vi "Command Engine.vi"(8 "error in (no error)":errorcluster, 10 "Parameters":T1 {"Config"."Industrial Settings"."Write Refs"."Data Reference" format="%.0x"; "Config"."Industrial Settings"."Read Refs"."Data Reference" format="%.0x"; "Config"."PID Settings"."Read Refs"."Data Reference" format="%.0x"; "Config"."PID Settings"."Write Refs"."Data Reference" format="%.0x"}, 11 "State Variables":T9) -> (0 "error out":errorcluster)   [LabVIEW 2015, in "Control Addon Engine.lvlib"]
uses:
  Control Addon Engine.lvlib
  Types/Network Engine State Variables.ctl
  <vilib>/NI/NI VeriStand Inline Async API/_VS Inline Async API/Process/Process.lvclass
  <vilib>/NI/VeriStand Addon Network Comm/Engine/VeriStand Comm.lvclass
  Types/RT Configuration.ctl
  Shared/Types/Gain Schedule.ctl
  Shared/Types/Compiled Settings.ctl
  Shared/Types/Compiled PID Settings.ctl
  <vilib>/NI Veristand/Custom Device API/Block Data Reference.ctl
  <vilib>/NI Veristand/Custom Device API/Data Reference.ctl
  Shared/Types/Compiled Industrial Settings.ctl
  Shared/Types/Compiled Industrial Parameters.ctl
  <vilib>/NI/VeriStand Addon Network Comm/Engine/VeriStand Comm.lvclass/VeriStand Comm.ctl
  Shared/Types/Update Parameters Message.ctl
  <vilib>/NI/NI VeriStand Inline Async API/_VS Inline Async API/Process/Process.lvclass/Process.ctl
  <vilib>/NI/NI VeriStand Inline Async API/_VS Inline Async API/Error Handling Process/SubVIs/Error.ConvertArray.vi
  <vilib>/NI/AMC/Read Next Message.vi
  <vilib>/NI/Tools/Keyed Array/Index.vi
  <vilib>/NI/AMC/Send Local Message.vi
  <vilib>/NI/AMC/Read Termination Message.vi
  <vilib>/NI/Tools/Keyed Array/Map String.vi
  <vilib>/NI/AMC/Create Single Message.vi
  <vilib>/NI/AMC/Update Message Routing Info.vi
  <vilib>/NI/Tools/String/Get Case Matching.vi
  <vilib>/NI/AMC/Send Message.vi
  <vilib>/NI/AMC/Globals.vi
  <vilib>/NI/VeriStand Addon Network Comm/Shared/Comm Constants.vi
  Shared/Control Addon Shared.lvlib
  <vilib>/NI VeriStand/Custom Device API/Custom Device API.lvlib
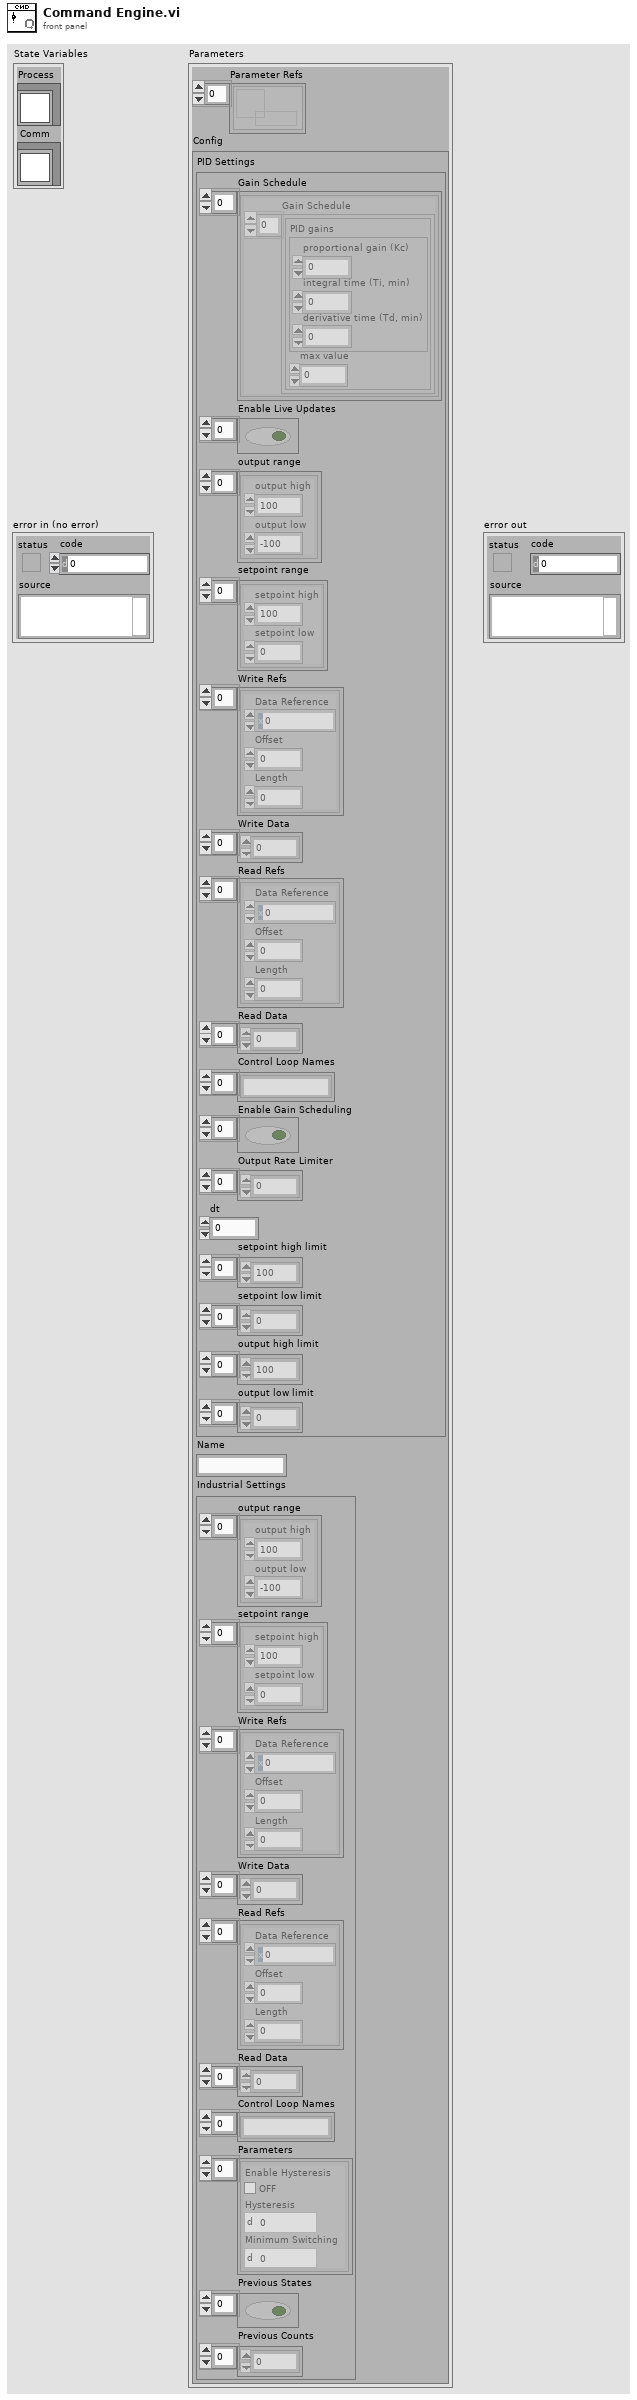
[diagram p1: front panel]
types:
  T1 = typedef "Control Addon Engine.lvlib/RT Configuration.ctl" = cluster{"Parameter Refs":refnum<data-value>[], "Config":T2}
  T2 = typedef "Control Addon Shared.lvlib/Compiled Settings.ctl" = cluster{"PID Settings":T3, "Name":string, "Industrial Settings":T7}
  T3 = typedef "Control Addon Shared.lvlib/Compiled PID Settings.ctl" = cluster{"Gain Schedule":T4[], "Enable Live Updates":bool[], "output range":cluster{"output high":dbl, "output low":dbl}[], "setpoint range":cluster{"setpoint high":dbl, "setpoint low":dbl}[], "Write Refs":T5[], "Write Data":dbl[], "Read Refs":T5[], "Read Data":dbl[], "Control Loop Names":string[], "Enable Gain Scheduling":bool[], "Output Rate Limiter":dbl[], "dt":dbl, "setpoint high limit":dbl[], "setpoint low limit":dbl[], "output high limit":dbl[], "output low limit":dbl[]}
  T4 = typedef "Control Addon Shared.lvlib/Gain Schedule.ctl" = cluster{"Gain Schedule":cluster{"PID gains":cluster{"proportional gain (Kc)":dbl, "integral time (Ti, min)":dbl, "derivative time (Td, min)":dbl}, "max value":dbl}[]}
  T5 = typedef "Custom Device API.lvlib/Block Data Reference.ctl" = cluster{"Data Reference":T6, "Offset":u64, "Length":u64}
  T6 = typedef "Custom Device API.lvlib/Data Reference.ctl" = i32
  T7 = typedef "Control Addon Shared.lvlib/Compiled Industrial Settings.ctl" = cluster{"output range":cluster{"output high":dbl, "output low":dbl}[], "setpoint range":cluster{"setpoint high":dbl, "setpoint low":dbl}[], "Write Refs":T5[], "Write Data":dbl[], "Read Refs":T5[], "Read Data":dbl[], "Control Loop Names":string[], "Parameters":T8[], "Previous States":bool[], "Previous Counts":u64[]}
  T8 = typedef "Control Addon Shared.lvlib/Compiled Industrial Parameters.ctl" = cluster{"Enable Hysteresis":bool, "Hysteresis":dbl, "Minimum Switching":u64}
  T9 = typedef "Control Addon Engine.lvlib/Network Engine State Variables.ctl" = cluster{"Process":refnum<class "Process.lvclass">, "Comm":refnum<class "VeriStand Comm.lvclass">}
  T10 = typedef "Control Addon Shared.lvlib/Update Parameters Message.ctl" = cluster{"Control Loop":string, "Gain Schedule":cluster{"PID gains":cluster{"proportional gain (Kc)":dbl, "integral time (Ti, min)":dbl, "derivative time (Td, min)":dbl}, "max value":dbl}[]}
  T11 = typedef "NI VeriStand Addon Network Comm.lvlib/VeriStand Comm.lvclass/Response Information.ctl" = cluster{"response name":string, "responseQ":string}
  T12 = typedef "Control Addon Shared.lvlib/Get Settings Message.ctl" = cluster{"Control Loop Names":string[], "Enable Live Updates":bool[], "Gain Schedule":T4[], "Enable Gain Scheduling":bool[]}
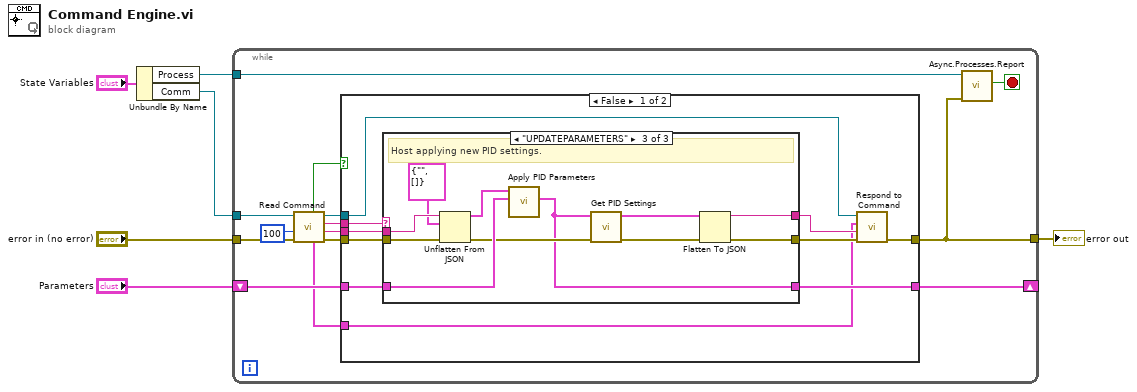
[diagram p0: block diagram]
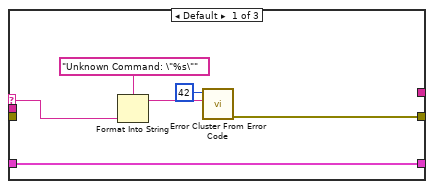
[diagram p2: hidden frame]
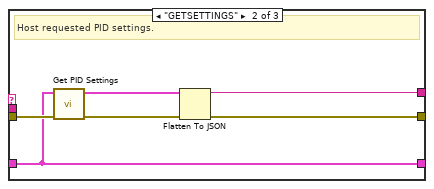
[diagram p3: hidden frame]
diagram:
  n1 = Unbundle By Name("State Variables") -> ("Process"=w3:refnum<class "Process.lvclass">, "Comm"=w1:refnum<class "VeriStand Comm.lvclass">)
  n2 = while {
    tunnel: "error in (no error)" -> [w18]
    tunnel: [w12] -> w4
    shift-right: [w19] -> _
    shift-left: "Parameters" -> [w20]
    tunnel: w3 -> [w16]
    tunnel: w1 -> [w10]
    stop <- w15 stop-if-true
    n3 = call <vilib>:"Read Command.vi"("error in (no error)"=w18, "timeout (100 ms)"=100 ("timeout (1 ms)"), "VeriStand Comm in"=w10) -> ("error out"=w17:errorcluster, "message value"=w13:string, "message name"=w11:string, "VeriStand Comm out"=w9:refnum<class "VeriStand Comm.lvclass">, "ResponseInfo"=w8:T11, "timed out?"=w7:bool)  [unwired: 3 in]
    n4 = case shown="False" w7 {
      tunnel: w20 -> [w30 w55]
      tunnel: [w29 w55] -> w19
      tunnel: w17 -> [w28 w54]
      tunnel: w13 -> [w27 _]
      tunnel: [w25 w54] -> w12
      tunnel: w11 -> [w23 _]
      tunnel: w9 -> [w22 _]
      tunnel: w8 -> [w21 _]
      frame False {
        n5 = case shown="\"UPDATEPARAMETERS\"" w23 {
          selector: w23 -> [w31 _ _]
          tunnel: w28 -> [_ w42 w47]
          tunnel: [w32 w38 w45] -> w26
          tunnel: w27 -> [_ _ w52]
          tunnel: w30 -> [w36 w41 w53]
          tunnel: [w36 w41 w49] -> w29
          tunnel: [_ w37 w43] -> w24
          frame Default {
            n6 = Format Into String(format string="Unknown Command: \"%s\"", w31) -> (resulting string=w33:string)  [unwired: 2 in, 1 out]
            n7 = call <vilib>:"Error Cluster From Error Code.vi"("error message (\"\")"=w33, "error code (0)"=42) -> ("error out"=w32:errorcluster)  [unwired: 7 in]
          }
          frame "GETSETTINGS" {
            # "Host requested PID settings."
            n8 = call "Get PID Settings.vi"("error in (no error)"=w42, "Parameters"=w41) -> ("error out"=w39:errorcluster, "PID Settings"=w40:T12)  [unwired: 8 in]
            n9 = Flatten To JSON(anything=w40, error in (no error)=w39) -> (JSON string=w37:string, 11:w38:errorcluster)  [unwired: 1 in]
          }
          frame "UPDATEPARAMETERS" {
            # "Host applying new PID settings."
            n10 = Unflatten From JSON(JSON string=w52, type and defaults=T10 {"Control Loop"="", "Gain Schedule"=[]}, error in (no error)=w47) -> (value=w51:T10, error out=w50:errorcluster)  [unwired: 4 in]
            n11 = call "Apply PID Parameters.vi"("Parameters in"=w53, "UpdateParameters"=w51) -> ("Parameters out"=w49:T1)  [unwired: 9 in]
            n12 = call "Get PID Settings.vi"("error in (no error)"=w50, "Parameters"=w49) -> ("error out"=w46:errorcluster, "PID Settings"=w44:T12)  [unwired: 8 in]
            n13 = Flatten To JSON(anything=w44, error in (no error)=w46) -> (JSON string=w43:string, 11:w45:errorcluster)  [unwired: 1 in]
          }
        }
        n14 = call <vilib>:"Respond to Command.vi"("error in (no error)"=w26, "message value"=w24, "ResponseInfo"=w21, "VeriStand Comm in"=w22) -> ("error out"=w25:errorcluster)  [unwired: 5 in, 2 out]
      }
      frame True {
      }
    }
    n15 = call <vilib>:"Async.Processes.Report.vi"("Error"=w12, "Process in"=w16) -> ("Stop"=w15:bool)  [unwired: 8 in, 1 out]
  }
  "error out" <- w4
